vi "Update Append View Value.vi"(5 "Display State In":T4={"Current Channels Info"=[], "Help Prefix"="", "Max Display Size"=8, "Max Size"=8, "Show Buttons"=TRUE, "Data Valid"=refnum, "Show Range"=FALSE, "Range Items"=[], "Range Index"=[]} caption="State", 7 "Channels In":T1, 11 "Channels Reference":refnum<vi>) -> ()   [LabVIEW 2021, in "myRIO Channel List.xctl"]
uses:
  <vilib>/myRIO/Common/Express VI Framework/xctls/myRIO Channel List/myRIO Channel List.xctl
  <vilib>/myRIO/Common/Express VI Framework/xctls/myRIO Channel List/State.ctl
  <vilib>/myRIO/Common/Profile Manager Framework/typedefs/Channel Info.ctl
  <vilib>/myRIO/Common/Express VI Framework/typedefs/Data Validate Ref.ctl
  <vilib>/myRIO/Common/Express VI Framework/xctls/myRIO Channel List/Data.ctl
  <vilib>/myRIO/Common/Express VI Framework/xctls/myRIO Channel List/typedefs/Channel Data.ctl
  <vilib>/myRIO/Common/Express VI Framework/xctls/myRIO Channel List/typedefs/Remove Channel.ctl
  <vilib>/myRIO/Common/Express VI Framework/xctls/myRIO Channel List/typedefs/Channel View.ctl
  <vilib>/myRIO/Common/Express VI Framework/xctls/myRIO Channel List/typedefs/Error Icon.ctl
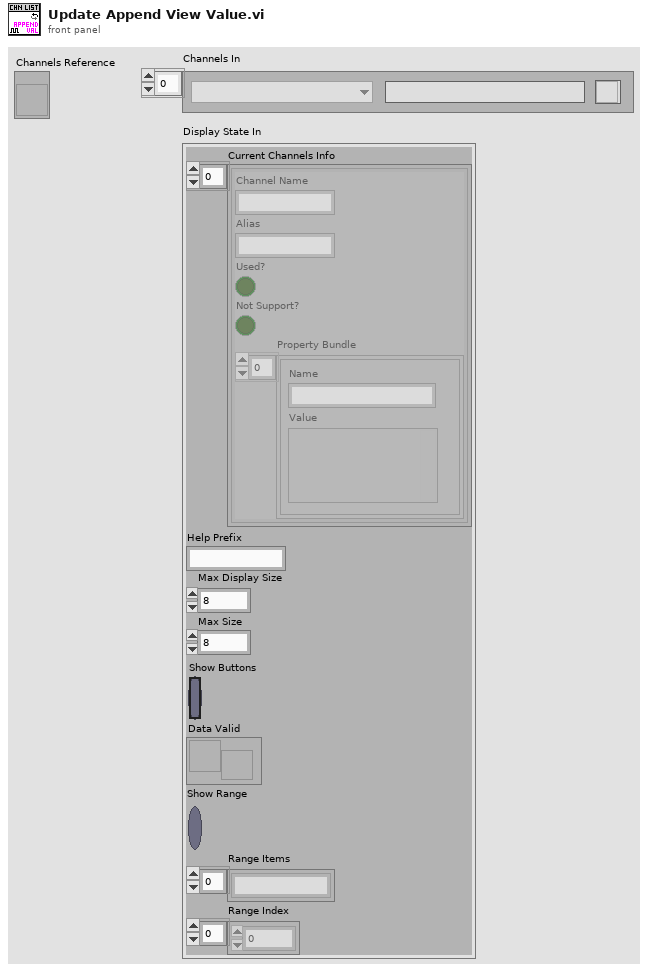
[diagram p1: front panel]
types:
  T1 = typedef "myRIO Channel List.xctl/Data.ctl" = T2[]
  T2 = typedef "myRIO Channel List.xctl/Channel Data.ctl" = cluster{"Channel Name":u16, "Channel Alias":string, "Remove Channel":T3, "Index":i32}
  T3 = typedef "myRIO Channel List.xctl/Remove Channel.ctl" = bool
  T4 = typedef "myRIO Channel List.xctl/State.ctl" = cluster{"Current Channels Info":T5[], "Help Prefix":string, "Max Display Size":i32, "Max Size":i32, "Show Buttons":bool, "Data Valid":T6, "Show Range":bool, "Range Items":string[], "Range Index":i32[]}
  T5 = typedef "Channel Info.ctl" = cluster{"Channel Name":string, "Alias":string, "Used?":bool, "Not Support?":bool, "Property Bundle":cluster{"Name":string, "Value":variant}[]}
  T6 = typedef "Data Validate Ref.ctl" = refnum<user-event>
  T7 = typedef "myRIO Channel List.xctl/Channel View.ctl" = cluster{"Error Icon":T8, "Channel Name":string, "Channel Alias":string, "Remove Channel":T3, "Index":i32, "Range":i32}
  T8 = typedef "myRIO Channel List.xctl/Error Icon.ctl" = bool
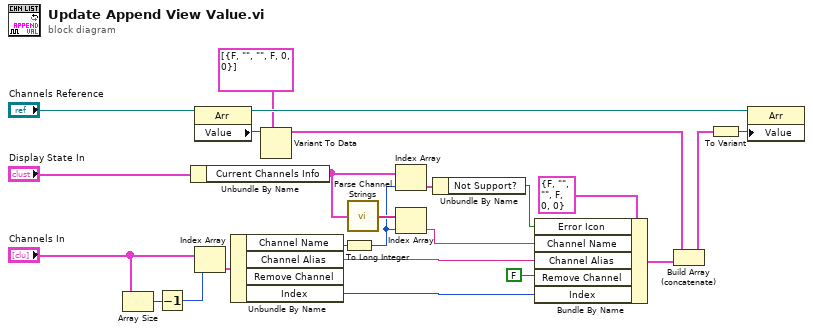
[diagram p0: block diagram]
diagram:
  n1 = Array Size(array="Channels In") -> (size(s)=w2:i32)
  n2 = Decrement(x=w2) -> (x-1=w1:i32)
  n3 = Unbundle By Name("Display State In") -> ("Current Channels Info"=w18:T5[])
  n4 = property class="Arr"(reference="Channels Reference") -> (reference out=w23:refnum<vi>, "Value"=w22:variant)  [unwired: 1 in, 1 out]
  n5 = Index Array(array="Channels In", index=w1) -> (element=w9:T2)
  n6 = Unbundle By Name(w9) -> ("Channel Name"=w15:u16, "Channel Alias"=w16:string, "Index"=w17:i32)  [unwired: 1 out]
  n7 = Variant To Data(type=T7[] [{"Error Icon"=FALSE, "Channel Name"="", "Channel Alias"="", "Remove Channel"=FALSE, "Index"=0, "Range"=0}], Variant=w22) -> (data=w5:T7[])  [unwired: 1 in, 1 out]
  n8 = To Long Integer(number=w15) -> (32bit integer=w13:i32)
  n9 = call <vilib>:"Parse Channel Strings.vi"("Channels Info"=w18) -> ("Channel Strings"=w20:string[])
  n10 = Index Array(array=w18, index=w13) -> (element=w11:T5)
  n11 = Index Array(array=w20, index=w13) -> (element=w14:string)
  n12 = Unbundle By Name(w11) -> ("Not Support?"=w12:bool)
  n13 = Bundle By Name(cluster=T7 {"Error Icon"=FALSE, "Channel Name"="", "Channel Alias"="", "Remove Channel"=FALSE, "Index"=0, "Range"=0} ("Channel"), "Error Icon"=w12, "Channel Name"=w14, "Channel Alias"=w16, "Remove Channel"=T3 FALSE, "Index"=w17) -> (w7:T7)
  n14 = Build Array (concatenate)(w5, w7) -> (w4:T7[])
  n15 = To Variant(anything=w4) -> (Variant=w8:variant)
  n16 = property class="Arr"(reference=w23, "Value"=w8) -> ()  [unwired: 1 in, 2 out]
